vi "create new vi.vi"(8 "error in":errorcluster, 11 "Show VI":bool=TRUE) -> (0 "error out":errorcluster, 3 "vi id":string)   [LabVIEW 2020]
doc: "Creates a new LabVIEW VI and shows the block diagram to the user. Use the returned vi id with other tools to modify the VI. Show VI usually should be set to true to show the user the newly created VI."
uses:
  G-AI Core/G-AI Core.lvlib
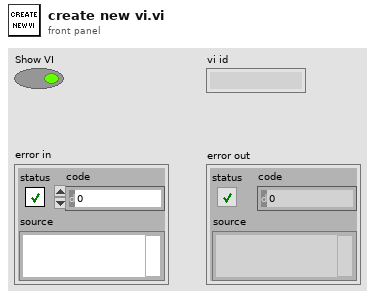
[diagram p1: front panel]
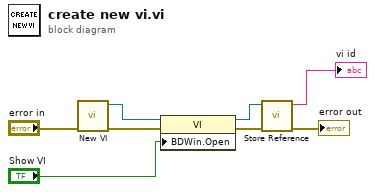
[diagram p0: block diagram]
diagram:
  n1 = call "New VI.vi"("error in"="error in") -> ("error out"=w8:errorcluster, "VI Refnum"=w7:refnum<vi>)  [unwired: 9 in]
  n2 = property class="VI"(reference=w7, error in=w8, "BDWin.Open"="Show VI") -> (reference out=w4:refnum<vi>, error out=w5:errorcluster)
  n3 = call "Store Reference.vi"("error in"=w5, "Reference"=w4) -> ("error out"=→"error out":errorcluster, "id"=→"vi id":string)  [unwired: 8 in]
